vi "Configure Bus Controller.vi"(7 "Virtual Memory Unit in":refnum<class "Virtual Memory Unit.lvclass">, 8 "error in (no error)":errorcluster, 11 "Bus Controller in":refnum<class "Bus Controller.lvclass">) -> (0 "error out":errorcluster, 3 "Bus Controller out":refnum<class "Bus Controller.lvclass">, 5 "Virtual Memory Unit out":refnum<class "Virtual Memory Unit.lvclass">)   [LabVIEW 2020, in "BCI-1553 API.lvlib" / "Bus Controller.lvclass"]
doc: "Builds all the configuration details specific to this Bus Controller. Major Frames, Minor Frames, and Messages are handled as a part of the instruction list construction."
uses:
  Bus Controller.lvclass
  Dependencies/Virtual Memory Unit/Virtual Memory Unit.lvclass
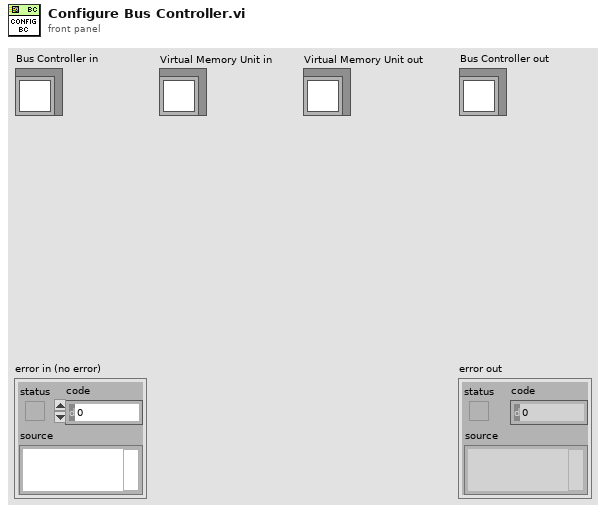
[diagram p1: front panel]
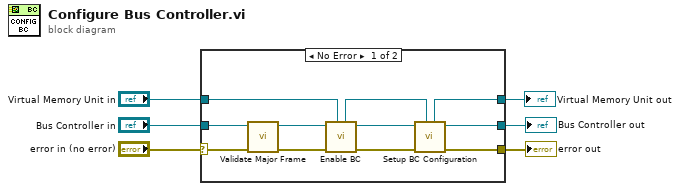
[diagram p0: block diagram]
diagram:
  n1 = case shown="No Error" "error in (no error)" {
    selector: "error in (no error)" -> [w11 w20]
    tunnel: [w15 w20] -> w5
    tunnel: [w16 w19] -> w3
    tunnel: "Bus Controller in" -> [w13 w19]
    tunnel: [w14 w18] -> w2
    tunnel: "Virtual Memory Unit in" -> [w17 w18]
    frame No Error {
      n2 = call "Validate Major Frame.vi"("error in (no error)"=w11, "Bus Controller in"=w13) -> ("error out"=w10:errorcluster, "Bus Controller out"=w12:refnum<class "Bus Controller.lvclass">)  [unwired: 8 in]
      n3 = call "Enable BC.vi"("Virtual Memory Unit in"=w17, "error in (no error)"=w10, "Bus Controller in"=w12) -> ("error out"=w7:errorcluster, "Bus Controller out"=w8:refnum<class "Bus Controller.lvclass">, "Virtual Memory Unit out"=w9:refnum<class "Virtual Memory Unit.lvclass">)  [unwired: 6 in]
      n4 = call "Setup BC Configuration.vi"("Virtual Memory Unit in"=w9, "error in (no error)"=w7, "Bus Controller in"=w8) -> ("error out"=w15:errorcluster, "Bus Controller out"=w16:refnum<class "Bus Controller.lvclass">, "Virtual Memory Unit out"=w14:refnum<class "Virtual Memory Unit.lvclass">)  [unwired: 6 in]
    }
    frame Error {
    }
  }
  "error out" <- w5
  "Bus Controller out" <- w3
  "Virtual Memory Unit out" <- w2
